vi "File-with-date-time-DONE.vi"(3 "error in (no error)":errorcluster) -> (8 "refnum out":refnum<file>)   [LabVIEW 2013]
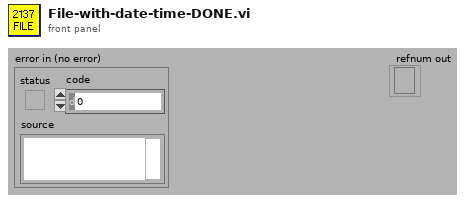
[diagram p1: front panel]
types:
  T1 = enum16{"open", "replace", "create", "open or create", "replace or create", "replace or create with confirmation"}
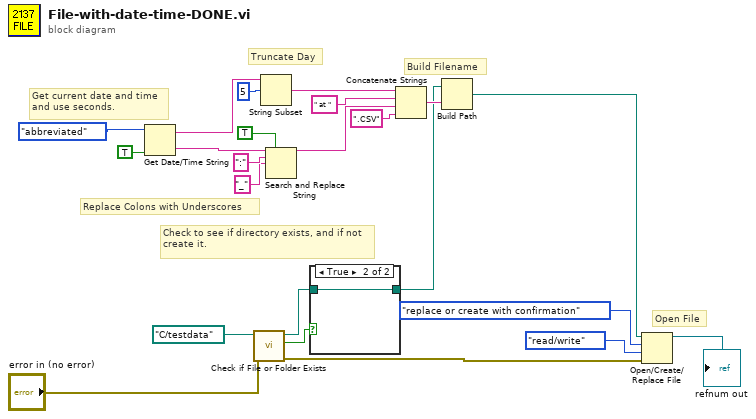
[diagram p0: block diagram]
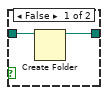
[diagram p2: hidden frame]
diagram:
  # "Open File"
  # "Build Filename"
  # "Replace Colons with Underscores"
  # "Truncate Day"
  # "Check to see if directory exists, and if not create it."
  # "Get current date and time\nand use seconds."
  n1 = Get Date/Time String(date format (0)=enum16{"short", "long", "abbreviated"}."abbreviated", want seconds? (F)=TRUE) -> (date string=w11:string, time string=w18:string)  [unwired: 1 in]
  n2 = call <vilib>:"Check if File or Folder Exists.vi"("error in (no error)"="error in (no error)", "path"=path "C:/testdata" ("path (use dialog)")) -> ("error out"=w3:errorcluster, "file or folder exists?"=w6:bool, "dup path"=w5:path)  [unwired: 7 in]
  n3 = String Subset(string=w11, offset (0)=5) -> (substring=w9:string)  [unwired: 1 in]
  n4 = Search and Replace String(replace all?=TRUE ("replace all? (F)"), input string=w18, search string=":", replace string="_" ("replace string (\"\")")) -> (result string=w13:string)  [unwired: 4 in, 3 out]
  n5 = case shown="True" w6 {
    tunnel: w5 -> [w25 w26]
    tunnel: [w24 w26] -> w4
    frame False {
      n6 = Create Folder(path (use dialog)=w25) -> (created path=w24:path)  [unwired: 2 in, 2 out]
    }
    frame True {
    }
  }
  n7 = Concatenate Strings(w9, " at " ("string"), w13, ".CSV" ("string")) -> (w20:string)
  n8 = Build Path(base path=w4, name or relative path=w20) -> (appended path=w19:path)
  n9 = Open/Create/Replace File(file path (use dialog)=w19, error in=w3, operation (0:open)=T1."replace or create with confirmation", access (0:read/write)=enum16{"read/write", "read-only", "write-only"}."read/write") -> (refnum out=→"refnum out":refnum<file>)  [unwired: 4 out]
